vi "Get Property.vi"(10 "Ctl Ref":refnum<vi>, 11 "Visible UIP In":refnum<class "VisibleUIP.lvclass">) -> (0 "Error Out":errorcluster, 3 "Visible UIP Out":refnum<class "VisibleUIP.lvclass">)   [LabVIEW 2020, in "UIM.lvlib" / "VisibleUIP.lvclass"]
uses:
  VisibleUIP.lvclass
  VisibleUIP.lvclass/VisibleUIP.ctl
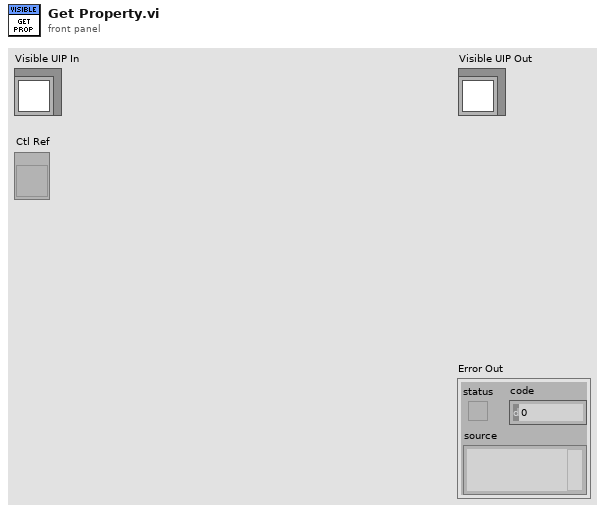
[diagram p1: front panel]
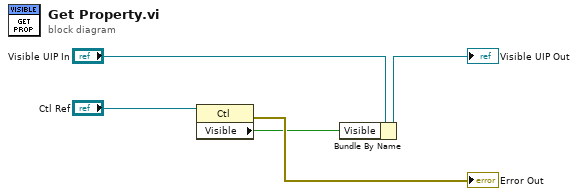
[diagram p0: block diagram]
diagram:
  n1 = property class="Ctl"(reference="Ctl Ref") -> (error out=→"Error Out":errorcluster, "Visible"=w2:bool)  [unwired: 1 in, 1 out]
  n2 = Bundle By Name(cluster="Visible UIP In", "Visible"=w2) -> (→"Visible UIP Out":refnum<class "VisibleUIP.lvclass">)
